vi "ServerStart.vi"(8 "error in (no error)":errorcluster, 11 "TcpServer in":refnum<class "TcpServer.lvclass">) -> (0 "error out":errorcluster, 3 "TcpServer out":refnum<class "TcpServer.lvclass">)   [LabVIEW 2022 SP3, in "TcpServer.lvlib" / "TcpServer.lvclass"]
uses:
  TcpServer.lvclass
  C:/Program Files (x86)/National Instruments/LabVIEW 2022/vi.lib/ActorFramework/Actor/Actor.lvclass
  C:/Users/jakub/repos/gh/sw4sys/lv-tcp-server-sample/LoggingActor/Source/LoggingActor/LoggingActor/LoggingActor.lvclass
  <vilib>/ActorFramework/Actor/Actor.lvclass/Actor.ctl
  <vilib>/ActorFramework/Message Enqueuer/Message Enqueuer.lvclass/Message Enqueuer.ctl
  LoggingActor/Source/LoggingActor/LoggingActor/LoggingActor.lvclass/LoggingActor.ctl
  TcpServer.lvclass/TcpServer.ctl
  _ServerState.ctl
  TcpSocket/Source/TcpSocket/TcpSocket/TcpSocket.lvclass/TcpSocket.ctl
  TcpSocket/Source/TcpSocket/TcpServer/TcpServer.lvclass/TcpServer.ctl
  TcpSocket/Source/TcpSocket/TcpSocket/Read Address.vi
  TcpSocket/Source/TcpSocket/TcpSocket/Read Port.vi
  TcpSocket/Source/TcpSocket/TcpSocket/Read Connection.vi
  TcpSocket/Source/TcpSocket/TcpSocket/Read ReadMode.vi
  TcpSocket/Source/TcpSocket/TcpSocket/Read OpenTimeout.vi
  TcpSocket/Source/TcpSocket/TcpSocket/Read ReadTimeout.vi
  TcpSocket/Source/TcpSocket/TcpSocket/Read WriteTimeout.vi
  TcpSocket/Source/TcpSocket/TcpServer/Read ConnectionTimeout.vi
  LoggingActor/Source/LoggingActor/LoggingActor/Read Logger.vi
  <vilib>/ActorFramework/Message Enqueuer/Init from Existing Queue.vi
  TcpSocket/Source/TcpSocket/TcpServer/TcpServer.lvclass
  C:/Users/jakub/repos/gh/sw4sys/lv-tcp-server-sample/TcpSocket/Source/TcpSocket/TcpSocket/TcpSocket.lvclass
  <vilib>/ActorFramework/Message Enqueuer/Message Enqueuer.lvclass
  Logger/Source/Logger/Logger.lvclass
  <vilib>/ActorFramework/Actor/Actor.lvclass
  TcpServer Messages/WaitForConnection Msg/WaitForConnection Msg.lvclass
  C:/Program Files (x86)/National Instruments/LabVIEW 2022/vi.lib/ActorFramework/Message/Message.lvclass
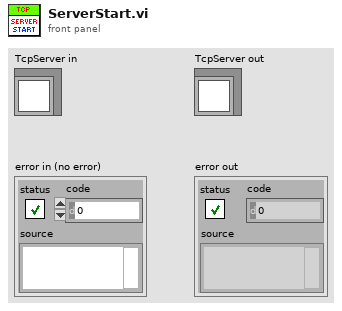
[diagram p1: front panel]
types:
  T1 = typedef "TcpServer.lvlib/TcpServer.lvclass/_ServerState.ctl" = enum16{"Idle", "Running"}
  T2 = enum16{"Standard", "Buffered", "CRLF", "Immediate"}
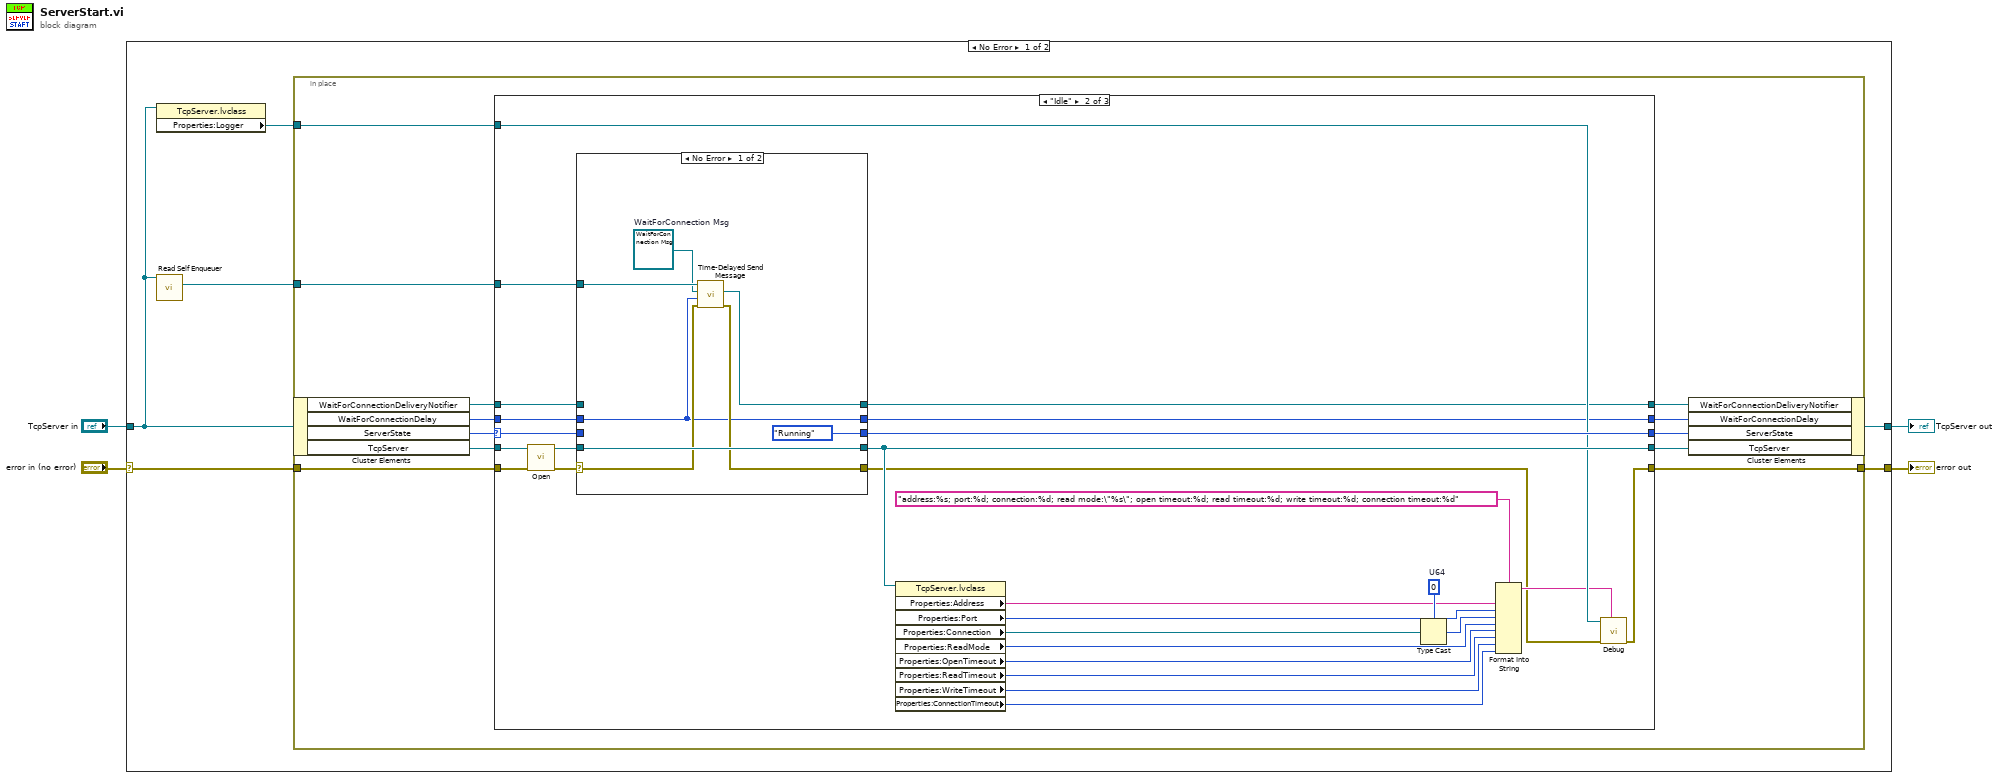
[diagram p0: block diagram]
diagram:
  n1 = case shown="No Error" "error in (no error)" {
    selector: "error in (no error)" -> [w10 w74]
    tunnel: [w8 w74] -> w3
    tunnel: [w7 w73] -> w1
    tunnel: "TcpServer in" -> [w6 w73]
    frame No Error {
      n2 = property class="TcpServer.lvclass"(reference=w6) -> ("Properties:Logger"=w5:refnum<class "Logger.lvclass">)  [unwired: 1 in, 2 out]
      n3 = call <vilib>:"Read Self Enqueuer.vi"("Actor"=w6) -> ("Self Enqueuer"=w9:refnum<class "Message Enqueuer.lvclass">)  [unwired: 10 in]
      n4 = in-place {
        in-place-border: [w22] -> w8
        in-place-border: w10 -> [w21]
        in-place-border: w9 -> [w16]
        in-place-border: w5 -> [w15]
        n5 = in-place-cluster #1(w6) -> ("WaitForConnectionDeliveryNotifier"=w13:refnum<notifier>, "WaitForConnectionDelay"=w14:i32, "ServerState"=w18:T1, "TcpServer"=w20:refnum<class "TcpServer.lvclass">)
        n6 = case shown="\"Idle\"" w18 {
          selector: w18 -> [w25 w49 w70]
          tunnel: [w26 w37 w71] -> w22
          tunnel: w21 -> [w26 w54 w71]
          tunnel: w20 -> [w27 w53 w72]
          tunnel: [w27 w39 w72] -> w19
          tunnel: [w25 w50 w70] -> w17
          tunnel: w16 -> [_ w48 _]
          tunnel: w15 -> [_ w36 _]
          tunnel: w14 -> [w23 w31 w68]
          tunnel: w13 -> [w24 w28 w69]
          tunnel: [w24 w30 w69] -> w12
          tunnel: [w23 w29 w68] -> w11
          frame Default {
          }
          frame "Idle" {
            w45 = u64 0  # U64
            n7 = call-dynamic "Open.vi"("error in (no error)"=w54, "TcpServer In"=w53) -> ("error out"=w52:errorcluster, "TcpServer Out"=w51:refnum<class "TcpServer.lvclass">)  [unwired: 8 in]
            n8 = case shown="No Error" w52 {
              selector: w52 -> [w59 w66]
              tunnel: [w58 w66] -> w34
              tunnel: [w62 w67] -> w39
              tunnel: w51 -> [w62 w67]
              tunnel: [_ServerState."Running" ("ServerState") w65] -> w50
              tunnel: w49 -> [_ w65]
              tunnel: w48 -> [w60 _]
              tunnel: w31 -> [w56 w63]
              tunnel: [w57 w64] -> w30
              tunnel: w28 -> [_ w64]
              tunnel: [w56 w63] -> w29
              frame No Error {
                w55 = refnum<class "WaitForConnection Msg.lvclass"> refnum  # WaitForConnection Msg
                n9 = call <vilib>:"Time-Delayed Send Message.vi"("error in (no error)"=w59, "Milliseconds To Wait"=w56, "Message"=w55, "Message Enqueuer"=w60) -> ("error out"=w58:errorcluster, "Delivery Notifier"=w57:refnum<notifier>)  [unwired: 6 in]
              }
              frame Error {
              }
            }
            n10 = property class="TcpServer.lvclass"(reference=w39) -> ("Properties:Address"=w33:string, "Properties:Port"=w32:u16, "Properties:Connection"=w47:refnum<k5>, "Properties:ReadMode"=w44:T2, "Properties:OpenTimeout"=w43:i32, "Properties:ReadTimeout"=w42:i32, "Properties:WriteTimeout"=w41:i32, "Properties:ConnectionTimeout"=w40:i32)  [unwired: 1 in, 2 out]
            n11 = Type Cast(type=w45, x=w47) -> (*(type *) &x=w46:u64)
            n12 = Format Into String(format string="address:%s; port:%d; connection:%d; read mode:\"%s\"; open timeout:%d; read timeout:%d; write timeout:%d; connection timeout:%d", w33, w32, w46, w44, w43, w42, w41, w40) -> (resulting string=w35:string)  [unwired: 2 in, 1 out]
            n13 = call-dynamic "Debug.vi"("Message"=w35, "error in (no error)"=w34, "Logger in"=w36) -> ("error out"=w37:errorcluster)  [unwired: 5 in, 1 out]
          }
          frame "Running" {
          }
        }
        n14 = in-place-cluster #1("WaitForConnectionDeliveryNotifier"=w12, "WaitForConnectionDelay"=w11, "ServerState"=w17, "TcpServer"=w19) -> (w7:refnum<class "TcpServer.lvclass">)
      }
    }
    frame Error {
    }
  }
  "error out" <- w3
  "TcpServer out" <- w1
